vi "Cal2-GetMode.vi"(8 "Calibration.vi running as top level VI?":bool, 10 "Mode in":T1, 11 "Path in":path) -> (1 "data mode":enum16{"Take new data point", "Refit Curve"}(ring), 2 "Mode out":T1, 3 "Boolean":bool)   [LabVIEW 2016]
uses:
  Anemometry Sub Vis/Calibration/Calib_mode.ctl
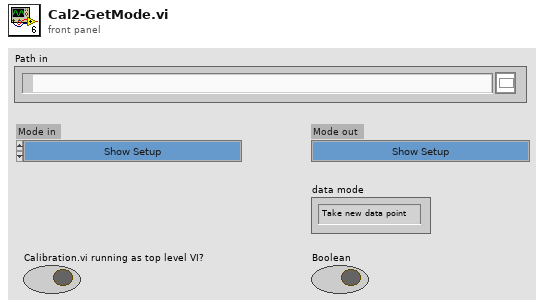
[diagram p1: front panel]
types:
  T1 = typedef "Calib_mode.ctl" = enum16{"Show Setup", "Take a New Calibration Point", "Refit Curve", "Setup Front Panel"}
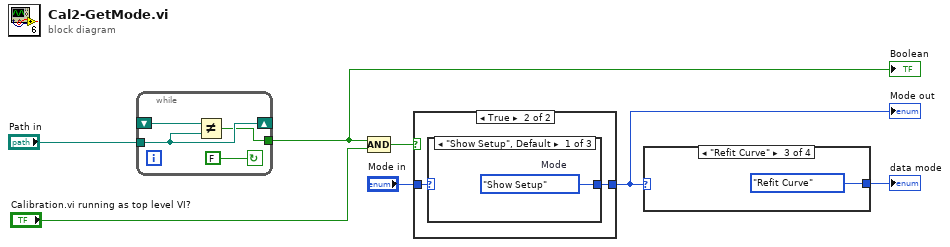
[diagram p0: block diagram]
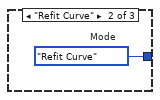
[diagram p3: hidden frame]
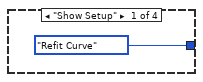
[diagram p5: hidden frame]
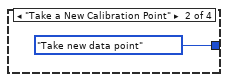
[diagram p6: hidden frame]
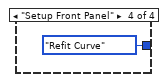
[diagram p7: hidden frame]
diagram:
  n1 = while {
    shift-right: [w10] -> _
    shift-left: _ -> [w11]
    tunnel: "Path in" -> [w10]
    tunnel: [w9] -> w4
    stop <- FALSE continue-if-true
    n2 = Not Equal?(x=w11, y=w10) -> (x != y?=w9:bool)
  }
  "Boolean" <- w4
  n3 = Compound Arithmetic op=AND(w4, "Calibration.vi running as top level VI?") -> (w5:bool)
  n4 = case shown="True" w5 {
    tunnel: "Mode in" -> [w12 w13]
    tunnel: [w12 w14] -> w7
    frame False {
    }
    frame True {
      n5 = case shown="\"Show Setup\", Default" w13 {
        selector: w13 -> [_ _ w17]
        tunnel: [w15 w16 w17] -> w14
        frame "Show Setup", Default {
          w15 = Calib_mode."Show Setup"  # Mode
        }
        frame "Refit Curve" {
          w16 = Calib_mode."Refit Curve"  # Mode
        }
        frame "Setup Front Panel" {
        }
      }
    }
  }
  "Mode out" <- w7
  n6 = case shown="\"Refit Curve\"" w7 {
    tunnel: [enum16{"Take new data point", "Refit Curve"}."Refit Curve" ("data mode") enum16{"Take new data point", "Refit Curve"}."Take new data point" ("data mode") enum16{"Take new data point", "Refit Curve"}."Refit Curve" ("data mode") enum16{"Take new data point", "Refit Curve"}."Refit Curve" ("data mode")] -> w2
    frame "Show Setup" {
    }
    frame "Take a New Calibration Point" {
    }
    frame "Refit Curve" {
    }
    frame "Setup Front Panel" {
    }
  }
  "data mode" <- w2
